vi "NI-Digital Burst I2C.vi"() -> ()   [LabVIEW 2023]
doc: "Overview\nDemonstrates how to use the NI-Digital Pattern Driver API to create and configure an instrument session and to burst a pattern on the digital pattern instrument using a start trigger."
uses:
  <instrlib>/niDigital/niDigital.llb/niDigital Selected Function.ctl
  <instrlib>/niDigital/niDigital.llb/niDigital Write Static Pin State.ctl
  <instrlib>/niDigital/niDigital.llb/niDigital Load Specifications Levels and Timing (Single).vi
  <instrlib>/niDigital/niDigital.llb/niDigital Data Mapping.ctl
  <instrlib>/Semi Device Control/Semiconductor Device Control.lvclass
  <instrlib>/Semi Device Control/Utils/DIO Pin State.ctl
  <instrlib>/niDigital/niDigital.llb/niDigital Write Source Waveform (Broadcast U32).vi
panel:
  in  "Tab Control":enum32{"SDC on", "Digital Low Level"}(tab)
  in  "Write?":bool
  in  "Register UID":string="CTRL_REG1"
  out "Register Value":u64
  in  "Write Value SDC":u64 format="%.0b"
  in  "Write":bool
  in  "Write Value":u64 format="%.0x"
  in  "Register Adress":u64 format="%.0x"
  out "Register Value Low Level":u64
  in  "Digital Pattern Resource":refnum<k15>="HSD_6571_C01_S02" caption="resource name"
  out "error out":errorcluster
  in  "Simulate?":bool
  # "Overview\nDemonstrates how to use the NI-Digital Pattern Driver API to create and configure an instrument session and to burst a pattern on the digital pattern instrument using a start trigger.\n\nInstructions\n1. Use the resource name control to select the digital pattern instrument. Ensure that the instrument name in the PinMap.pinmap file matches the resource name of the digital pattern instrument. The default value for the resource name is \"PXI1Slot2,PXI1Slot3\".\n2. Use the start trigger mode tab control to select the start trigger mode to use. The active tab determines the configured start trigger at run time. Some tabs include additional configuration options.\n3. Run the VI.\n4. To run on hardware deselect Simulate?  and modify the resource name as appropriate."
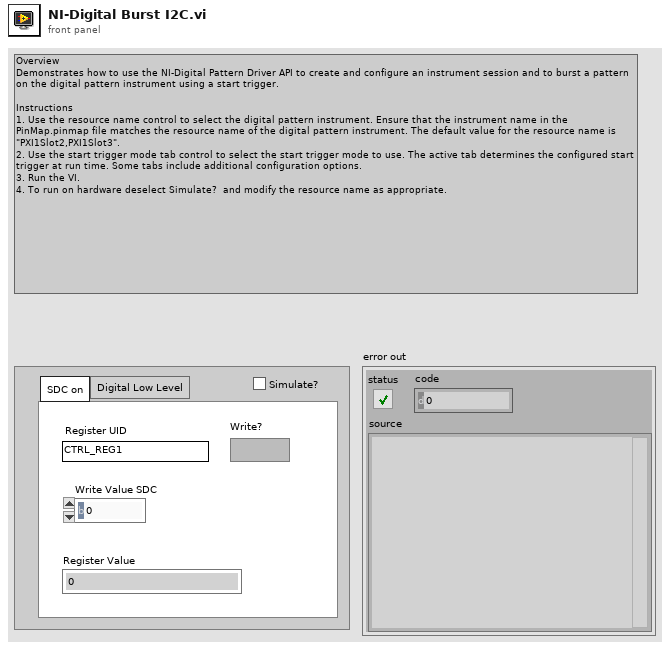
[diagram p1: front panel]
types:
  T1 = typedef "Semiconductor Device Control.lvclass/DIO Pin State.ctl" = enum16{"Low", "High", "Term"}
  T2 = typedef "niDigital Write Static Pin State.ctl" = u8
  T3 = typedef "niDigital Data Mapping.ctl" = i32
  T4 = typedef "niDigital Selected Function.ctl" = i32
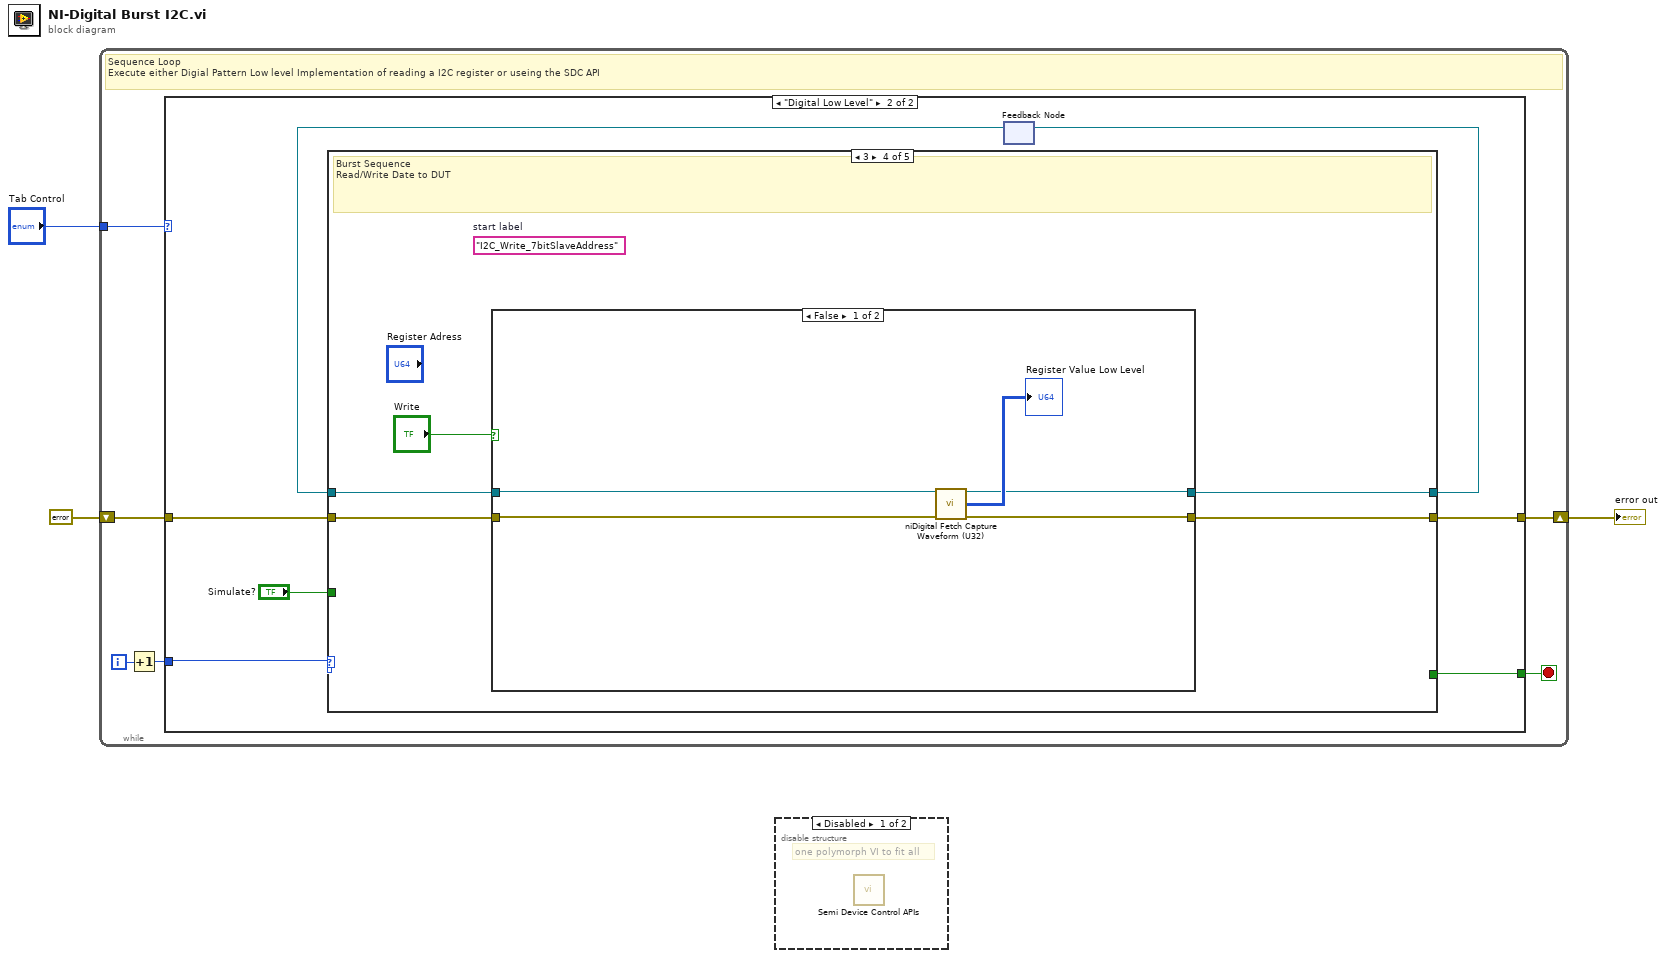
[diagram p0: block diagram]
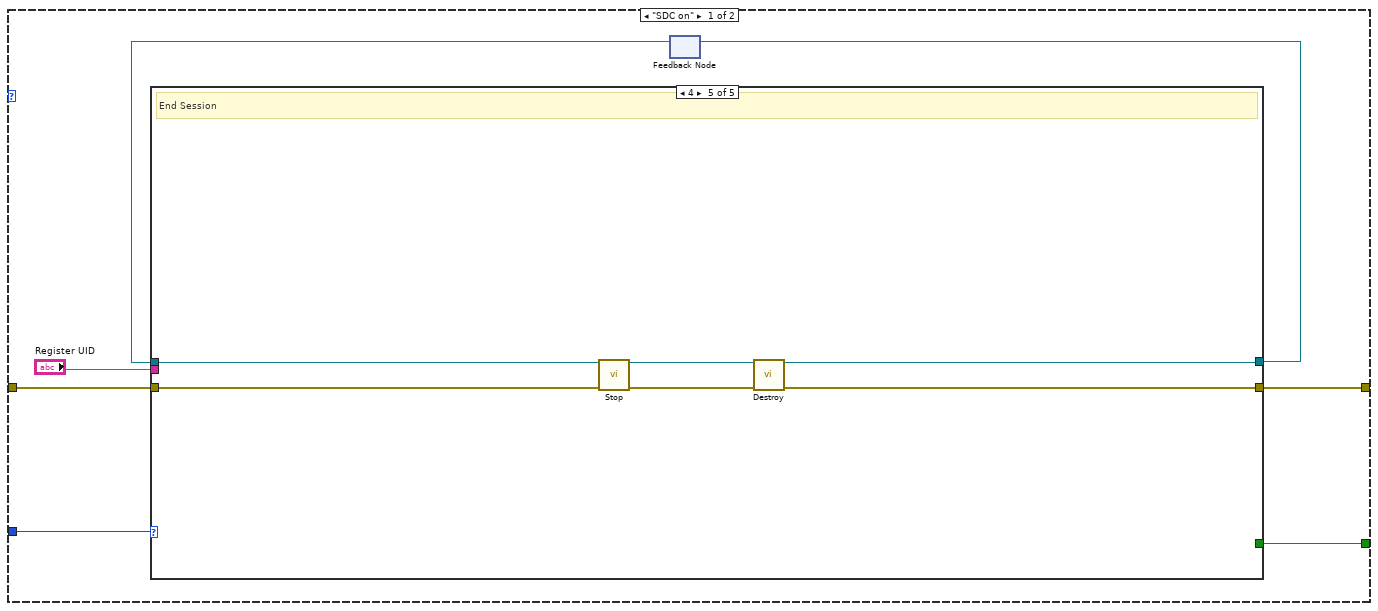
[diagram p3: hidden frame]
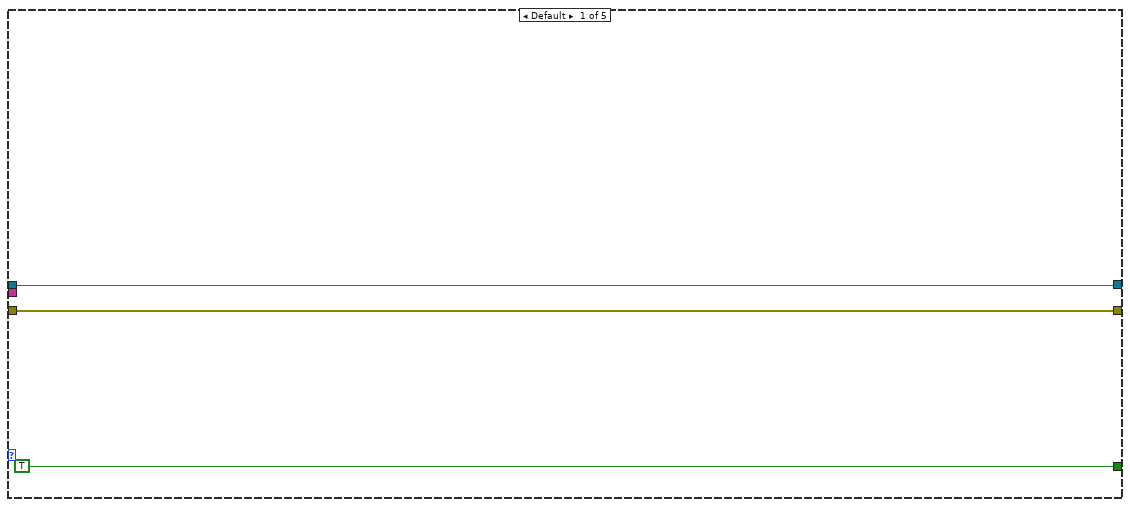
[diagram p4: hidden frame]
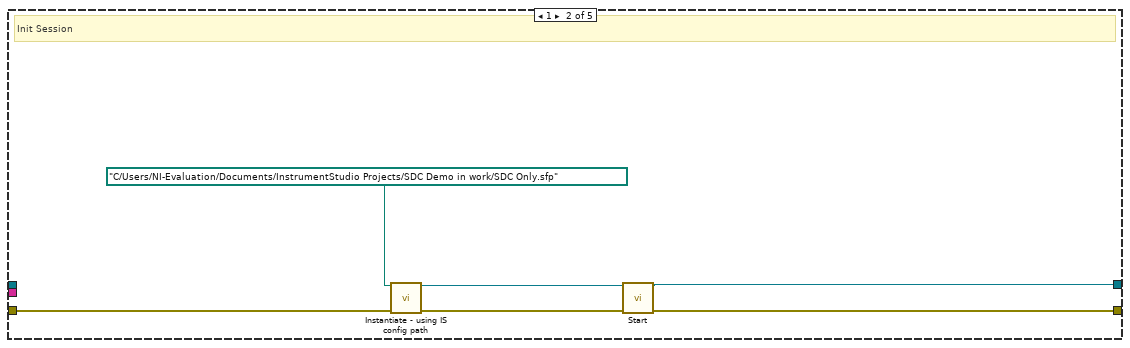
[diagram p5: hidden frame]
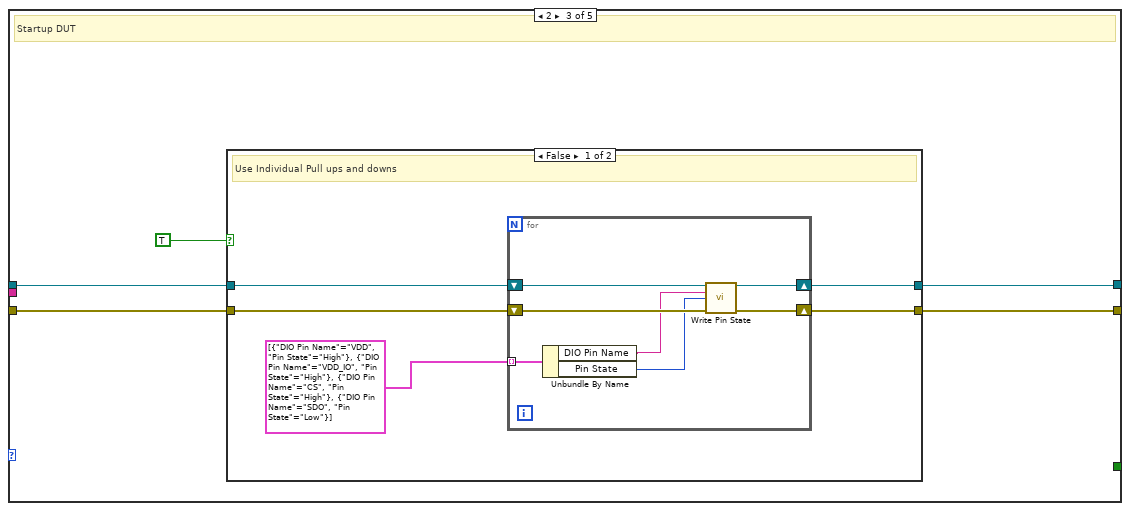
[diagram p6: hidden frame]
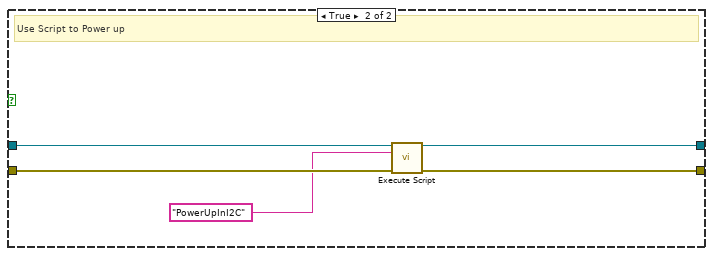
[diagram p7: hidden frame]
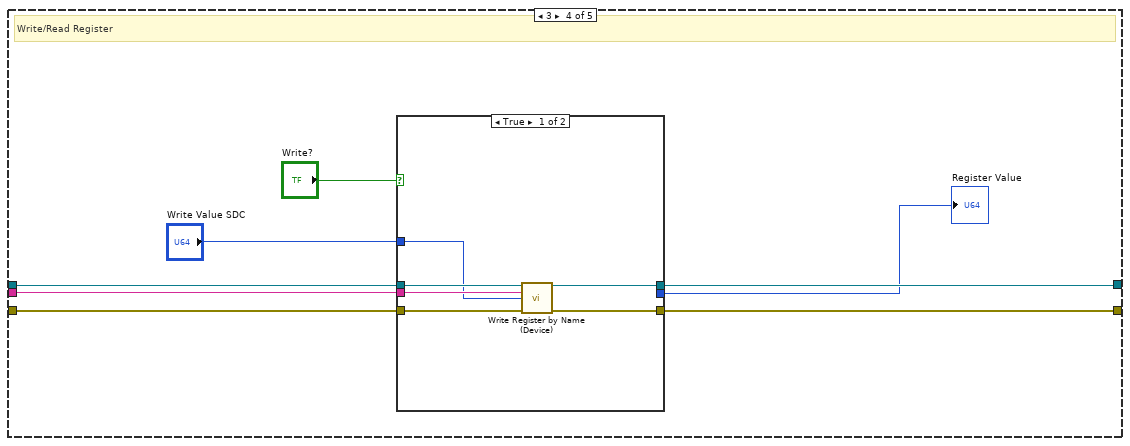
[diagram p8: hidden frame]
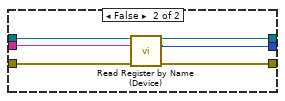
[diagram p9: hidden frame]
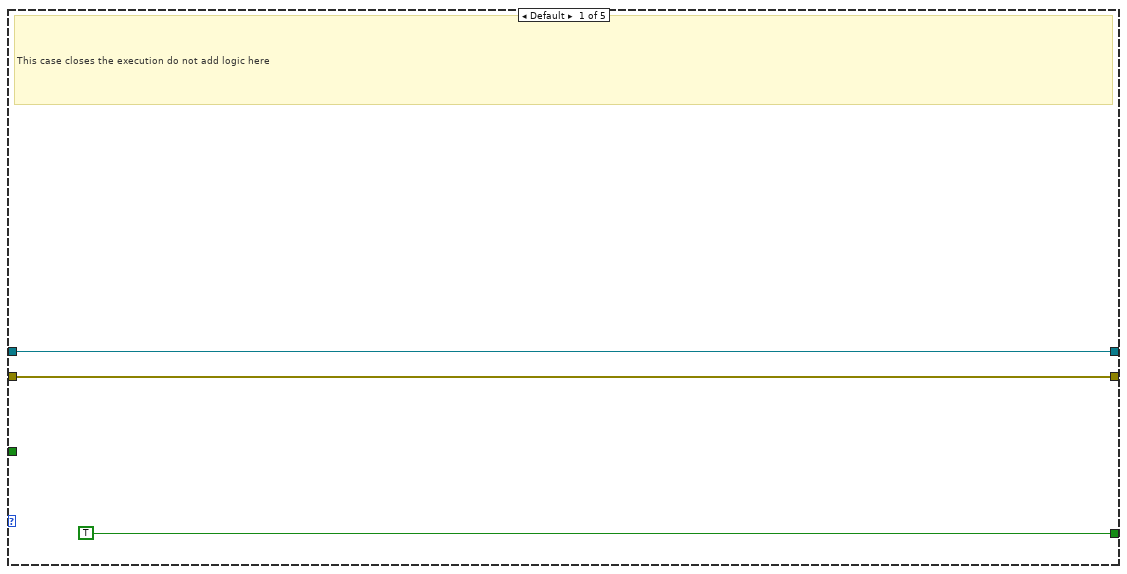
[diagram p10: hidden frame]
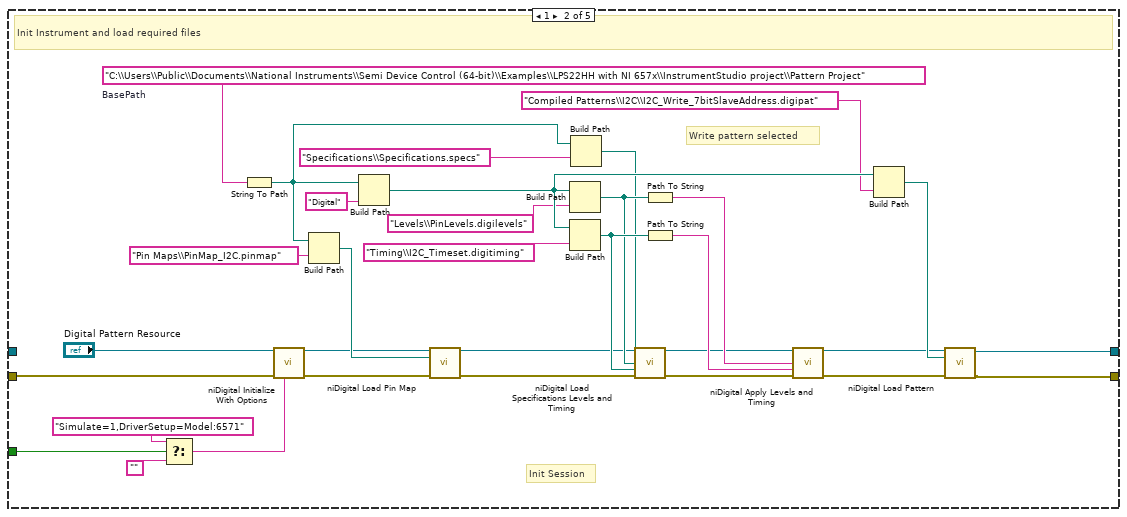
[diagram p11: hidden frame]
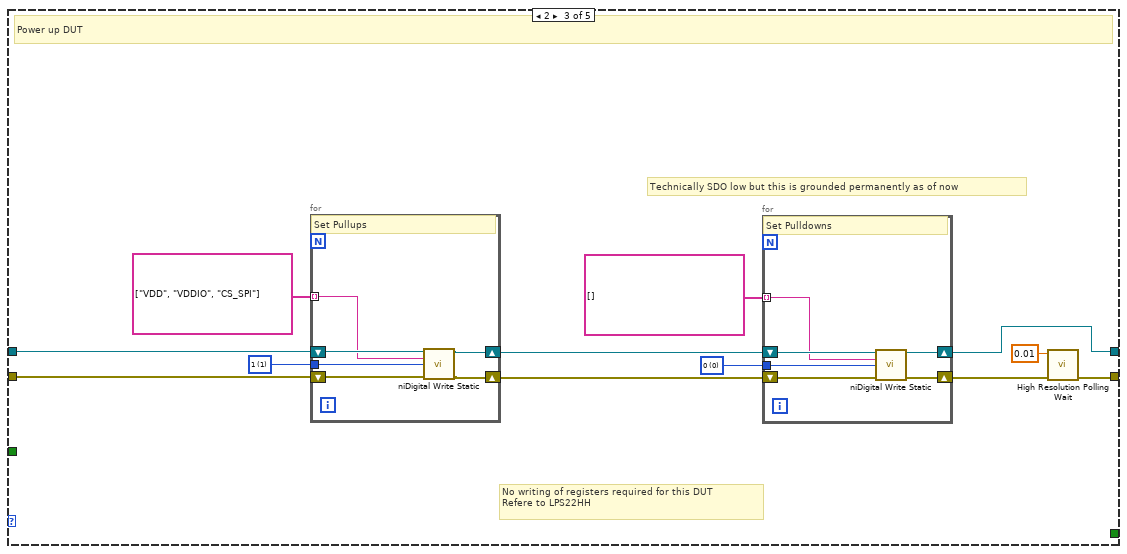
[diagram p12: hidden frame]
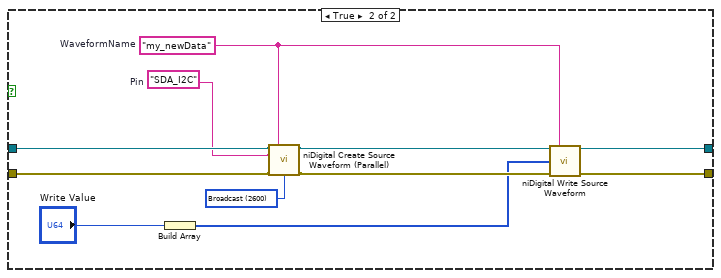
[diagram p13: hidden frame]
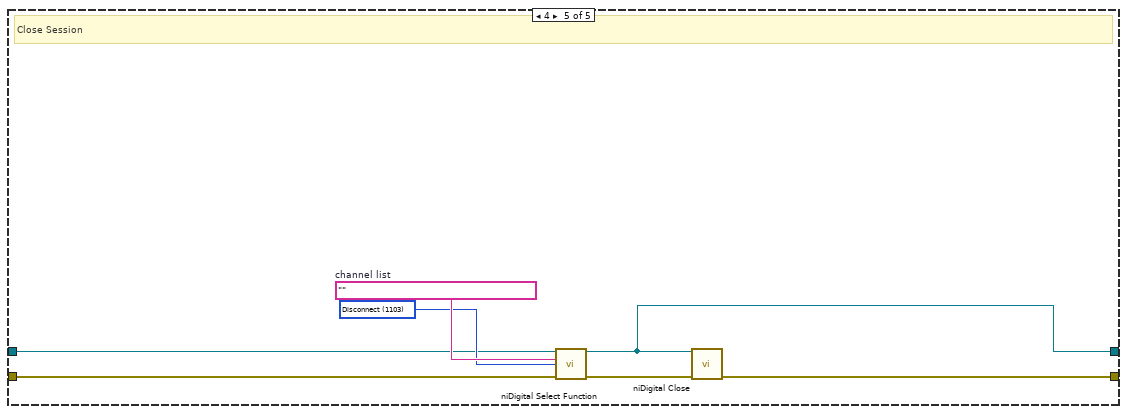
[diagram p14: hidden frame]
diagram:
  n1 = while {
    shift-right: [w8] -> w3
    shift-left: errorcluster {"status"=FALSE, "code"=0, "source"=""} ("error out") -> [w9]
    tunnel: "Tab Control" -> [w4]
    i -> [w6]
    stop <- w7 stop-if-true
    # "Sequence Loop\nExecute either Digial Pattern Low level Implementation of reading a I2C register or useing the SDC API"
    n2 = Increment(x=w6) -> (x+1=w5:i32)
    n3 = case shown="\"Digital Low Level\"" w4 {
      tunnel: w9 -> [w14 w80]
      tunnel: [w13 w79] -> w8
      tunnel: [w15 w78] -> w7
      tunnel: w5 -> [w16 w76]
      frame "SDC on" {
        n4 = feedback #1() -> (w11:refnum<class "Semiconductor Device Control.lvclass">)  [unwired: 1 in]
        n5 = case shown="4" w16 {
          tunnel: [TRUE _ _ _ _] -> w15
          tunnel: w14 -> [w18 w25 w30 w55 w71]
          tunnel: [w18 w22 w29 w54 w69] -> w13
          tunnel: w11 -> [w17 _ w28 w52 w70]
          tunnel: [w17 w21 w27 w53 w68] -> w12
          tunnel: "Register UID" -> [_ _ _ w51 _]
          frame Default {
          }
          frame 1 {
            # "Init Session"
            n6 = call <instrlib>:"Instantiate - using IS config path.vi"("IS Semi Device Control config path"=path "C:/Users/NI-Evaluation/Documents/InstrumentStudio Projects/SDC Demo in work/SDC Only.sfp", "error in (no error)"=w25) -> ("Device Control session out"=w24:refnum<class "Semiconductor Device Control.lvclass">, "error out"=w23:errorcluster)  [unwired: 12 in]
            n7 = call <instrlib>:"Start.vi"("Device Control session in"=w24, "error in (no error)"=w23) -> ("Device Control session out"=w21:refnum<class "Semiconductor Device Control.lvclass">, "error out"=w22:errorcluster)  [unwired: 12 in]
          }
          frame 2 {
            # "Startup DUT"
            n8 = case shown="False" TRUE {
              tunnel: w30 -> [w35 w47]
              tunnel: [w34 w46] -> w29
              tunnel: w28 -> [w33 w45]
              tunnel: [w32 w44] -> w27
              frame False {
                # "Use Individual Pull ups and downs"
                n9 = for {
                  shift-right: [w41] -> w34
                  shift-left: w35 -> [w42]
                  shift-right: [w39] -> w32
                  shift-left: w33 -> [w40]
                  tunnel: cluster{"DIO Pin Name":string, "Pin State":T1}[] [{"DIO Pin Name"="VDD", "Pin State"=enum."High"}, {"DIO Pin Name"="VDD_IO", "Pin State"=enum."High"}, {"DIO Pin Name"="CS", "Pin State"=enum."High"}, {"DIO Pin Name"="SDO", "Pin State"=enum."Low"}] -> [w38] mode=indexing
                  n10 = Unbundle By Name(w38) -> ("DIO Pin Name"=w37:string, "Pin State"=w36:T1)
                  n11 = call <instrlib>:"Write Pin State.vi"("Device Control session in"=w40, "DIO Pin Name"=w37, "Pin State"=w36, "error in (no error)"=w42) -> ("Device Control session out"=w39:refnum<class "Semiconductor Device Control.lvclass">, "error out"=w41:errorcluster)  [unwired: 10 in]
                }
              }
              frame True {
                # "Use Script to Power up"
                n12 = call <instrlib>:"Execute Script.vi"("Device Control session in"=w45, "Script Name"="PowerUpInI2C", "error in"=w47) -> ("Device Control session out"=w44:refnum<class "Semiconductor Device Control.lvclass">, "error out"=w46:errorcluster)  [unwired: 10 in, 1 out]
              }
            }
          }
          frame 3 {
            # "Write/Read Register"
            n13 = case shown="True" "Write?" {
              tunnel: w55 -> [w59 w67]
              tunnel: [w58 w66] -> w54
              tunnel: [w57 w65] -> w53
              tunnel: w52 -> [w61 w64]
              tunnel: w51 -> [w60 w63]
              tunnel: [_ w62] -> w50
              tunnel: "Write Value SDC" -> [w56 _]
              frame True {
                n14 = call <instrlib>:"Write Register by Name (Device).vi"("Device Control session in"=w61, "Register UID"=w60, "Register Data"=w56, "error in (no error)"=w59) -> ("Device Control session out"=w57:refnum<class "Semiconductor Device Control.lvclass">, "error out"=w58:errorcluster)  [unwired: 10 in]
              }
              frame False {
                n15 = call <instrlib>:"Read Register by Name (Device).vi"("Device Control session in"=w64, "Register UID"=w63, "error in (no error)"=w67) -> ("Device Control session out"=w65:refnum<class "Semiconductor Device Control.lvclass">, "Register Data"=w62:u64, "error out"=w66:errorcluster)  [unwired: 10 in]
              }
            }
            "Register Value" <- w50
          }
          frame 4 {
            # "End Session"
            n16 = call <instrlib>:"Stop.vi"("Device Control session in"=w70, "error in (no error)"=w71) -> ("Device Control session out"=w72:refnum<class "Semiconductor Device Control.lvclass">, "error out"=w73:errorcluster)  [unwired: 12 in]
            n17 = call <instrlib>:"Destroy.vi"("Device Control session in"=w72, "error in (no error)"=w73) -> ("Device Control session out"=w68:refnum<class "Semiconductor Device Control.lvclass">, "error out"=w69:errorcluster)  [unwired: 12 in]
          }
        }
        n18 = feedback-in #1(w12) -> ()
      }
      frame "Digital Low Level" {
        n19 = feedback #2() -> (w75:refnum<k15>)  [unwired: 1 in]
        n20 = case shown="3" w76 {
          tunnel: [w81 w84 w116 w144 w161] -> w74
          tunnel: w75 -> [w81 _ w126 w143 w163]
          tunnel: w80 -> [w82 w88 w127 w142 w164]
          tunnel: [w82 w86 w124 w141 w162] -> w79
          tunnel: [TRUE _ _ _ _] -> w78
          tunnel: "Simulate?" -> [_ w87 _ _ _]
          frame Default {
            # "This case closes the execution do not add logic here"
          }
          frame 1 {
            w92 = "C:\\Users\\Public\\Documents\\National Instruments\\Semi Device Control (64-bit)\\Examples\\LPS22HH with NI 657x\\InstrumentStudio project\\Pattern Project"  # BasePath
            # "Write pattern selected"
            # "Init Session"
            # "Init Instrument and load required files"
            n21 = Select(t="Simulate=1,DriverSetup=Model:6571", s=w87, f="") -> (s? t:f=w108:string)
            n22 = String To Path(string=w92) -> (path=w114:path)
            n23 = call <instrlib>:"niDigital Initialize With Options.vi"("resource name"="Digital Pattern Resource", "option string"=w108, "error in"=w88) -> ("instrument handle"=w103:refnum<k15>, "error out"=w104:errorcluster)  [unwired: 11 in]
            n24 = Build Path(base path=w114, name or relative path="Pin Maps\\PinMap_I2C.pinmap") -> (appended path=w109:path)
            n25 = Build Path(base path=w114, name or relative path="Digital") -> (appended path=w115:path)
            n26 = call <instrlib>:"niDigital Load Pin Map.vi"("instrument handle"=w103, "pin map file"=w109, "error in"=w104) -> ("instrument handle out"=w106:refnum<k15>, "error out"=w107:errorcluster)  [unwired: 11 in]
            n27 = Build Path(base path=w115, name or relative path="Levels\\PinLevels.digilevels") -> (appended path=w112:path)
            n28 = Build Path(base path=w115, name or relative path="Timing\\I2C_Timeset.digitiming") -> (appended path=w113:path)
            n29 = Build Path(base path=w114, name or relative path="Specifications\\Specifications.specs") -> (appended path=w111:path)
            n30 = call-poly <instrlib>:"niDigital Load Specifications Levels and Timing.vi"("instrument handle"=w106, "specifications file path"=w111, "levels file path"=w112, "timing file path"=w113, "error in"=w107) -> ("instrument handle out"=w98:refnum<k15>, "error out"=w99:errorcluster)  [unwired: 9 in]
            n31 = Path To String(path=w112) -> (string=w105:string)
            n32 = Path To String(path=w113) -> (string=w102:string)
            n33 = call <instrlib>:"niDigital Apply Levels and Timing.vi"("instrument handle"=w98, "levels sheet"=w105, "timing sheet"=w102, "error in"=w99) -> ("instrument handle out"=w101:refnum<k15>, "error out"=w100:errorcluster)  [unwired: 10 in]
            n34 = Build Path(base path=w115, name or relative path="Compiled Patterns\\I2C\\I2C_Write_7bitSlaveAddress.digipat") -> (appended path=w110:path)
            n35 = call <instrlib>:"niDigital Load Pattern.vi"("instrument handle"=w101, "pattern file"=w110, "error in"=w100) -> ("instrument handle out"=w84:refnum<k15>, "error out"=w86:errorcluster)  [unwired: 11 in]
          }
          frame 2 {
            w120 = T2 0 items=["0"=0, "1"=1, "X"=5] ("state")
            w125 = T2 1 items=["0"=0, "1"=1, "X"=5] ("state")
            # "Technically SDO low but this is grounded permanently as of now"
            # "No writing of registers required for this DUT\nRefere to LPS22HH"
            # "Power up DUT"
            n36 = for {
              tunnel: w125 -> [w137]
              tunnel: string[] ["VDD", "VDDIO", "CS_SPI"] ("channel list") -> [w136] mode=indexing
              shift-right: [w135] -> w119
              shift-left: w126 -> [w138]
              shift-right: [w134] -> w118
              shift-left: w127 -> [w139]
              # "Set Pullups"
              n37 = call <instrlib>:"niDigital Write Static.vi"("instrument handle"=w138, "channel list"=w136, "state"=w137, "error in"=w139) -> ("instrument handle out"=w135:refnum<k15>, "error out"=w134:errorcluster)  [unwired: 10 in]
            }
            n38 = for {
              tunnel: w120 -> [w131]
              tunnel: string[] [] ("channel list") -> [w130] mode=indexing
              shift-right: [w129] -> w117
              shift-left: w118 -> [w133]
              shift-right: [w128] -> w116
              shift-left: w119 -> [w132]
              # "Set Pulldowns"
              n39 = call <instrlib>:"niDigital Write Static.vi"("instrument handle"=w132, "channel list"=w130, "state"=w131, "error in"=w133) -> ("instrument handle out"=w128:refnum<k15>, "error out"=w129:errorcluster)  [unwired: 10 in]
            }
            n40 = call <vilib>:"High Resolution Polling Wait.vi"("error in (no error)"=w117, "seconds to wait"=0.01) -> ("error out"=w124:errorcluster)  [unwired: 9 in]
          }
          frame 3 {
            (unwired) "I2C_Write_7bitSlaveAddress"  # start label
            # "Burst Sequence\nRead/Write Date to DUT"
            n41 = case shown="False" "Write" {
              tunnel: [w145 w152] -> w144
              tunnel: w143 -> [w148 w160]
              tunnel: w142 -> [w147 w159]
              tunnel: [w146 w155] -> w141
              frame False {
                n42 = call <instrlib>:"niDigital Fetch Capture Waveform (U32).vi"("instrument handle"=w148, "error in"=w147) -> ("instrument handle out"=w145:refnum<k15>, "data"=→"Register Value Low Level":u32[][], "error out"=w146:errorcluster)  [unwired: 11 in]
              }
              frame True {
                w158 = "SDA_I2C"  # Pin
                w157 = T3 2600 items=["Broadcast"=2600, "Site Unique"=2601] ("data mapping")
                w151 = "my_newData"  # WaveformName
                n43 = Build Array("Write Value") -> (w150:u64[])
                n44 = call <instrlib>:"niDigital Create Source Waveform (Parallel).vi"("instrument handle"=w160, "waveform name"=w151, "data mapping"=w157, "pin list"=w158, "error in"=w159) -> ("instrument handle out"=w153:refnum<k15>, "error out"=w154:errorcluster)  [unwired: 9 in]
                n45 = call-poly <instrlib>:"niDigital Write Source Waveform.vi"("instrument handle"=w153, "waveform name"=w151, "waveform data"=w150, "error in"=w154) -> ("instrument handle out"=w152:refnum<k15>, "error out"=w155:errorcluster)  [unwired: 10 in]
              }
            }
          }
          frame 4 {
            w166 = ""  # channel list
            w165 = T4 1103 items=["Digital"=1100, "PPMU"=1101, "Off"=1102, "Disconnect"=1103] ("function")
            # "Close Session"
            n46 = call <instrlib>:"niDigital Select Function.vi"("instrument handle"=w163, "channel list"=w166, "function"=w165, "error in"=w164) -> ("instrument handle out"=w161:refnum<k15>, "error out"=w167:errorcluster)  [unwired: 10 in]
            n47 = call <instrlib>:"niDigital Close.vi"("instrument handle"=w161, "error in"=w167) -> ("error out"=w162:errorcluster)  [unwired: 13 in]
          }
        }
        n48 = feedback-in #2(w74) -> ()
      }
    }
  }
  "error out" <- w3
  n49 = disable-structure shown="Disabled" {
    frame Disabled {
      # "one polymorph VI to fit all"
      n50 = call-poly <instrlib>:"Semi Device Control APIs.vi"() -> ()  [unwired: 14 in, 2 out]
    }
    frame Enabled {
    }
  }
